vi "Do.vi"(8 "error in (no error)":errorcluster, 10 "Actor in":refnum<class "Actor.lvclass">, 11 "Write Beep Parameters Msg":refnum<class "Write Beep Parameters Msg.lvclass">) -> (0 "error out":errorcluster, 2 "Actor out":refnum<class "Actor.lvclass">)   [LabVIEW 2016, in "CS++BeepActor.lvlib" / "Write Beep Parameters Msg.lvclass"]
doc: "This VI delivers the message to the actor by calling the appropriate method(s) on the actor."
uses:
  Write Beep Parameters Msg.lvclass
  <vilib>/ActorFramework/Actor/Actor.lvclass
  C:/User/Brand/LVP/TASCA/UTCS/Packages/CSPP_Core/Actors/CS++PVMonitor Messages/CS++PVUpdate Msg/CS++PVUpdate Msg.lvclass
  Beep/Beep.lvclass
  C:/Program Files (x86)/National Instruments/LabVIEW 2016/vi.lib/ActorFramework/Actor/Actor.lvclass
  CSPP_Core/Actors/CS++PVMonitor Messages/CS++PVUpdate Msg/CS++PVUpdate Msg.lvclass/CS++PVUpdate Msg.ctl
  CSPP_Core/Classes/CS++ProcessVariables/ProcessVariable/PV.lvclass/PV.ctl
  Write Beep Parameters Msg.lvclass/Write Beep Parameters Msg.ctl
  CSPP_Core/Classes/CS++ProcessVariables/ProcessVariable/PV.lvclass
  CSPP_Core/Actors/CS++PVMonitor Messages/CS++PVUpdate Msg/CS++PVUpdate Msg.lvclass
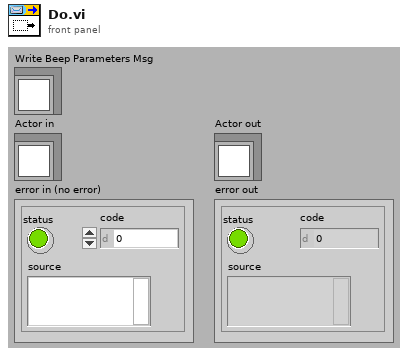
[diagram p1: front panel]
types:
  T1 = cluster{"Frequency (440)":dbl[unit], "Duration":dbl[unit], "Use System Alert?":bool}
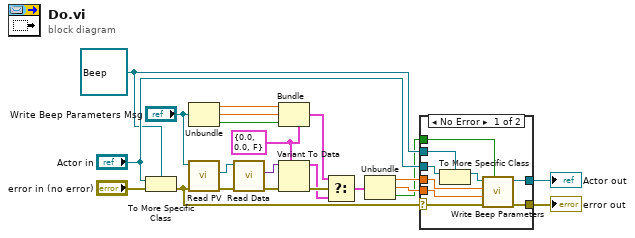
[diagram p0: block diagram]
diagram:
  w14 = T1 {"Frequency (440)"=0.0, "Duration"=0.0, "Use System Alert?"=FALSE} ("Type")
  w18 = refnum<class "Beep.lvclass"> refnum ("Actor in")
  n1 = To More Specific Class(target class=w18, reference="Actor in", error in="error in (no error)") -> (error out=w7:errorcluster)  [unwired: 1 out]
  n2 = Unbundle ("Pre-Unbundler")("Write Beep Parameters Msg") -> (w3:dbl[unit], w2:dbl[unit], w1:bool)
  n3 = call "Read PV.vi"("error in (no error)"=w7, "CS++PVUpdate Msg in"="Write Beep Parameters Msg") -> ("error out"=w17:errorcluster, "PV"=w13:refnum<class "PV.lvclass">)  [unwired: 7 in, 1 out]
  n4 = call "Read Data.vi"("error in (no error)"=w17, "PV in"=w13) -> ("error out"=w11:errorcluster, "Data"=w12:variant)  [unwired: 7 in, 1 out]
  n5 = Bundle ("Pre-Bundler")(cluster=w14, "Frequency (440)"=w3, "Duration"=w2, "Use System Alert?"=w1) -> (w15:T1)
  n6 = Variant To Data(error in=w11, type=w14, Variant=w12) -> (data=w9:T1, error out=w16:errorcluster)
  n7 = Select ("MainSelect")(t=w15, s=w16, f=w9) -> (s? t:f=w10:T1)
  n8 = Unbundle ("Main-Unbundler")(w10) -> ("Frequency (440)"=w6:dbl[unit], "Duration"=w5:dbl[unit], "Use System Alert?"=w4:bool)
  n9 = case shown="No Error" w7 {
    selector: w7 -> [w29 w33]
    tunnel: [w31 w33] -> w21
    tunnel: [w30 w32] -> w20
    tunnel: "Actor in" -> [w28 w32]
    tunnel: w18 -> [w27 _]
    tunnel: w6 -> [w25 _]
    tunnel: w5 -> [w24 _]
    tunnel: w4 -> [w23 _]
    frame No Error {
      n10 = To More Specific Class(target class=w27, reference=w28) -> (specific class reference=w26:refnum<class "Beep.lvclass">)  [unwired: 1 in, 1 out]
      n11 = call "Write Beep Parameters.vi"("Use System Alert?"=w23, "error in (no error)"=w29, "Duration"=w24, "Frequency (440)"=w25, "Beep in"=w26) -> ("error out"=w31:errorcluster, "Beep out"=w30:refnum<class "Beep.lvclass">)  [unwired: 5 in]
    }
    frame Error {
    }
  }
  "error out" <- w21
  "Actor out" <- w20
